vi "Write Alarm Limits.vi"(8 "error in":errorcluster, 10 "Alarm Limits":T1, 11 "PV Data in":refnum<class "PV Data.lvclass">) -> (0 "error out":errorcluster, 3 "PV Data out":refnum<class "PV Data.lvclass">)   [LabVIEW 2020, in "PV Access.lvlib" / "PV Data.lvlib" / "PV Data.lvclass"]
uses:
  PV Data.lvclass
  PV Data.lvclass/PV Data.ctl
  Write Field (Boolean).vi
  Write Field (Variant).vi
  Write Field (I32).vi
  Write Field (DBL).vi
  Alarm Severity.ctl
  PV Data.lvlib
  Alarm Limits.ctl
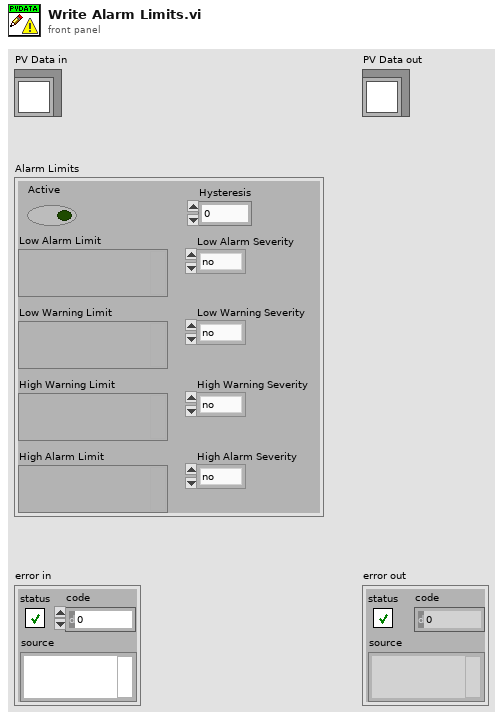
[diagram p1: front panel]
types:
  T1 = typedef "PV Access.lvlib/PV Data.lvlib/Alarm Limits.ctl" = cluster{"Active":bool, "Low Alarm Limit":variant, "Low Warning Limit":variant, "High Warning Limit":variant, "High Alarm Limit":variant, "Low Alarm Severity":T2, "Low Warning Severity":T2, "High Warning Severity ":T2, "High Alarm Severity":T2, "Hysteresis":dbl}
  T2 = typedef "PV Access.lvlib/PV Data.lvlib/Alarm Severity.ctl" = enum32{"no", "minor", "major", "record", "invalid", "undefined", ""}
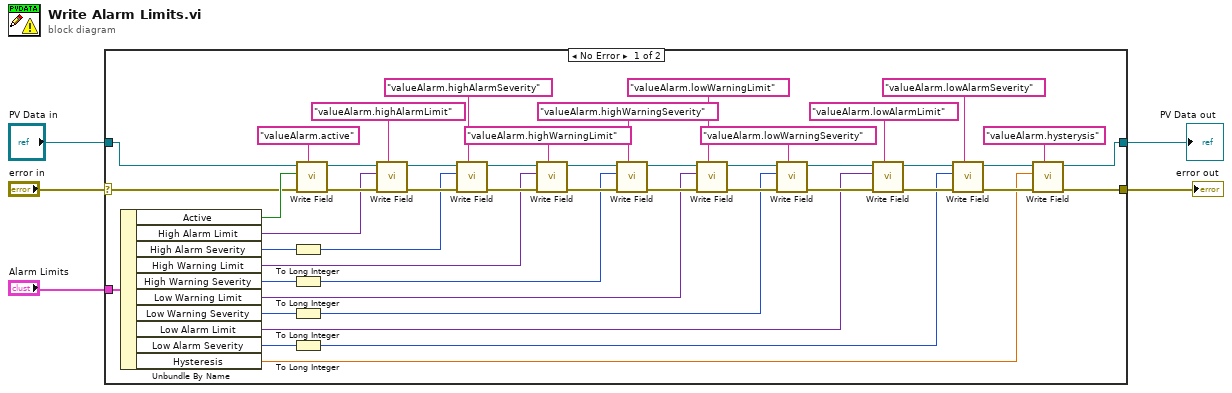
[diagram p0: block diagram]
diagram:
  n1 = case shown="No Error" "error in" {
    selector: "error in" -> [w9 w54]
    tunnel: [w6 w54] -> w5
    tunnel: "PV Data in" -> [w8 w53]
    tunnel: [w7 w53] -> w2
    tunnel: "Alarm Limits" -> [w24 _]
    frame No Error {
      n2 = Unbundle By Name(w24) -> ("Active"=w23:bool, "High Alarm Limit"=w22:variant, "High Alarm Severity"=w19:T2, "High Warning Limit"=w15:variant, "High Warning Severity"=w18:T2, "Low Warning Limit"=w13:variant, "Low Warning Severity"=w17:T2, "Low Alarm Limit"=w11:variant, "Low Alarm Severity"=w20:T2, "Hysteresis"=w21:dbl)
      n3 = To Long Integer(number=w19) -> (32bit integer=w16:i32)
      n4 = To Long Integer(number=w18) -> (32bit integer=w14:i32)
      n5 = To Long Integer(number=w17) -> (32bit integer=w12:i32)
      n6 = To Long Integer(number=w20) -> (32bit integer=w10:i32)
      n7 = call-poly "Write Field.vi"("field name"="valueAlarm.active", "error in"=w9, "value"=w23, "PV Data in"=w8) -> ("error out"=w51:errorcluster, "PV Data out"=w50:refnum<class "PV Data.lvclass">)  [unwired: 5 in, 1 out]
      n8 = call-poly "Write Field.vi"("field name"="valueAlarm.highAlarmLimit", "error in (no error)"=w51, "value in"=w22, "PV Data in"=w50) -> ("error out"=w42:errorcluster, "PV Data out"=w33:refnum<class "PV Data.lvclass">)  [unwired: 5 in, 1 out]
      n9 = call-poly "Write Field.vi"("field name"="valueAlarm.highAlarmSeverity", "error in"=w42, "value"=w16, "PV Data in"=w33) -> ("error out"=w43:errorcluster, "PV Data out"=w34:refnum<class "PV Data.lvclass">)  [unwired: 5 in, 1 out]
      n10 = call-poly "Write Field.vi"("field name"="valueAlarm.highWarningLimit", "error in (no error)"=w43, "value in"=w15, "PV Data in"=w34) -> ("error out"=w44:errorcluster, "PV Data out"=w35:refnum<class "PV Data.lvclass">)  [unwired: 5 in, 1 out]
      n11 = call-poly "Write Field.vi"("field name"="valueAlarm.highWarningSeverity", "error in"=w44, "value"=w14, "PV Data in"=w35) -> ("error out"=w45:errorcluster, "PV Data out"=w36:refnum<class "PV Data.lvclass">)  [unwired: 5 in, 1 out]
      n12 = call-poly "Write Field.vi"("field name"="valueAlarm.lowWarningLimit", "error in (no error)"=w45, "value in"=w13, "PV Data in"=w36) -> ("error out"=w46:errorcluster, "PV Data out"=w37:refnum<class "PV Data.lvclass">)  [unwired: 5 in, 1 out]
      n13 = call-poly "Write Field.vi"("field name"="valueAlarm.lowWarningSeverity", "error in"=w46, "value"=w12, "PV Data in"=w37) -> ("error out"=w47:errorcluster, "PV Data out"=w38:refnum<class "PV Data.lvclass">)  [unwired: 5 in, 1 out]
      n14 = call-poly "Write Field.vi"("field name"="valueAlarm.lowAlarmLimit", "error in (no error)"=w47, "value in"=w11, "PV Data in"=w38) -> ("error out"=w48:errorcluster, "PV Data out"=w39:refnum<class "PV Data.lvclass">)  [unwired: 5 in, 1 out]
      n15 = call-poly "Write Field.vi"("field name"="valueAlarm.lowAlarmSeverity", "error in"=w48, "value"=w10, "PV Data in"=w39) -> ("error out"=w41:errorcluster, "PV Data out"=w40:refnum<class "PV Data.lvclass">)  [unwired: 5 in, 1 out]
      n16 = call-poly "Write Field.vi"("field name"="valueAlarm.hysterysis", "error in"=w41, "value"=w21, "PV Data in"=w40) -> ("error out"=w6:errorcluster, "PV Data out"=w7:refnum<class "PV Data.lvclass">)  [unwired: 5 in, 1 out]
    }
    frame Error {
    }
  }
  "error out" <- w5
  "PV Data out" <- w2
